vi "Set Hardware Configuration File Path.vi"(8 "error in":errorcluster, 10 "hardware configuration file path":path, 11 "Ballard ARINC 429 custom device in":T1 format="%.0x") -> (0 "error out":errorcluster, 3 "Ballard ARINC 429 custom device out":T1 format="%.0x")   [LabVIEW 2020, in "AIM ARINC 429 Scripting.lvlib"]
doc: "Specifies the <b>hardware configuration file path</b>. The hardware configuration file is deployed to the RT target and must be consistent with system configuration for successful deployment and avionics bus communication."
uses:
  AIM ARINC 429 Scripting.lvlib
  <vilib>/NI VeriStand/Custom Device API/Custom Device Item Ref.ctl
  <vilib>/NI VeriStand/Custom Device API/Dependent File Optional Info.ctl
  Constants.vi
  <vilib>/NI VeriStand/Custom Device API/Set Item Property (Dependent File).vi
  <vilib>/NI VeriStand/Custom Device API/Custom Device API.lvlib
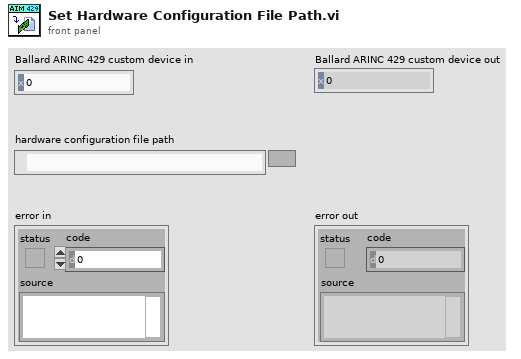
[diagram p1: front panel]
types:
  T1 = typedef "Custom Device API.lvlib/Custom Device Item Ref.ctl" = u64
  T2 = typedef "Custom Device API.lvlib/Dependent File Optional Info.ctl" = cluster{"Version":string, "RTDestination":path, "ForceDownload":bool, "SupportedTarget":string, "MD5":string}
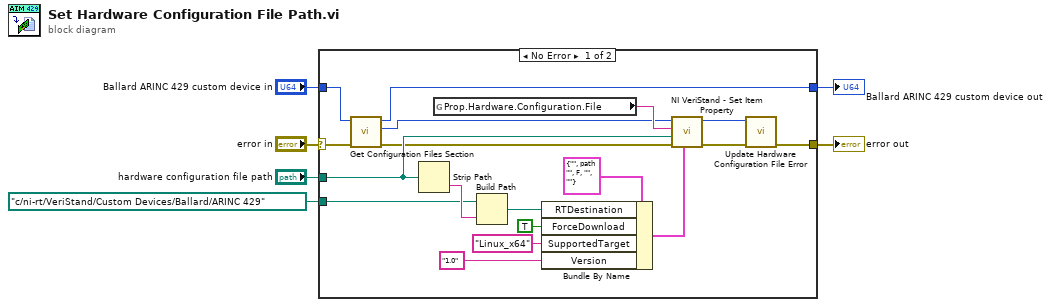
[diagram p0: block diagram]
diagram:
  n1 = case shown="No Error" "error in" {
    selector: "error in" -> [w11 w26]
    tunnel: "Ballard ARINC 429 custom device in" -> [w8 w25]
    tunnel: [w21 w26] -> w5
    tunnel: [w7 w25] -> w3
    tunnel: "hardware configuration file path" -> [w18 _]
    tunnel: path "c:/ni-rt/VeriStand/Custom Devices/Ballard/ARINC 429" ("RTDestination") -> [w16 _]
    frame No Error {
      n2 = call "Get Configuration Files Section.vi"("error in"=w11, "Custom device Ref"=w8) -> ("error out"=w10:errorcluster, "Configuration files Ref"=w9:T1, "Custom device Ref out"=w7:T1)  [unwired: 7 in]
      n3 = Strip Path(path=w18) -> (name=w17:string)  [unwired: 1 out]
      n4 = global read "Constants.vi" "Prop.Hardware.Configuration.File"() -> (w24:string)
      n5 = Build Path(base path=w16, name or relative path=w17) -> (appended path=w15:path)
      n6 = Bundle By Name(cluster=T2 {"Version"="", "RTDestination"=path "", "ForceDownload"=FALSE, "SupportedTarget"="", "MD5"=""} ("OptionalInfo"), "RTDestination"=w15, "ForceDownload"=TRUE, "SupportedTarget"="Linux_x64", "Version"="1.0") -> (w19:T2)
      n7 = call-poly <vilib>:"NI VeriStand - Set Item Property.vi"("OptionalInfo"=w19, "error in (no error)"=w10, "Path"=w18, "Property Name"=w24, "Item Ref in"=w9) -> ("error out"=w22:errorcluster, "Item Ref out"=w23:T1)  [unwired: 4 in, 1 out]
      n8 = call "Update Hardware Configuration File Error.vi"("error in"=w22, "Configuration files Ref"=w23) -> ("error out"=w21:errorcluster)  [unwired: 8 in, 1 out]
    }
    frame Error {
    }
  }
  "error out" <- w5
  "Ballard ARINC 429 custom device out" <- w3
